vi "Msg DeQ.vi"(11 "Msg Queue in":refnum<class "Msg Q.lvclass">) -> (0 "error out":errorcluster, 2 "Msg":refnum<class "Msg.lvclass">)   [LabVIEW 2021, in "LVCAM.lvlib" / "Msg Q.lvclass"]
uses:
  Msg Q.lvclass
  Msg/Msg.lvclass
  Msg Q.lvclass/Msg Q.ctl
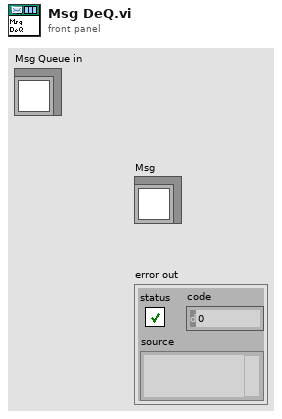
[diagram p1: front panel]
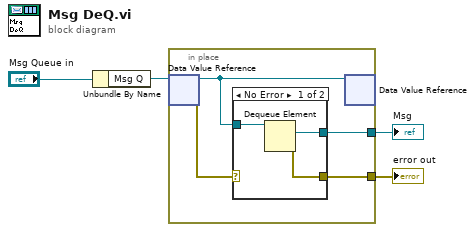
[diagram p0: block diagram]
diagram:
  n1 = Unbundle By Name("Msg Queue in") -> ("Msg Q"=w3:refnum<data-value>)
  n2 = in-place {
    in-place-border: [w7] -> w1
    in-place-border: [w6] -> w2
    n3 = in-place-dvr #1(w3) -> (w5:refnum<queue>, w8:errorcluster)
    n4 = case shown="No Error" w8 {
      selector: w8 -> [_ w12]
      tunnel: w5 -> [w11 _]
      tunnel: [w10 w12] -> w6
      tunnel: [w9 _] -> w7
      frame No Error {
        n5 = Dequeue Element(queue=w11) -> (element=w9:refnum<class "Msg.lvclass">, error out=w10:errorcluster)  [unwired: 2 in, 2 out]
      }
      frame Error {
      }
    }
    n6 = in-place-dvr #1(w5) -> ()  [unwired: 2 out]
  }
  "error out" <- w2
  "Msg" <- w1
